vi "Self-Test.vi"(8 "error in (no error)":errorcluster, 11 "VISA resource name":refnum<visa-resource-name>) -> (0 "error out":errorcluster, 1 "Self-Test Result Message":string, 2 "Self-Test Result Code":i32, 3 "VISA resource name out":refnum<visa-resource-name>)   [LabVIEW 2012, in "Micos_uic.lvlib"]
doc: "Runs the instrument's self-test routine and returns the test results."
uses:
  <instrlib>/Micos_uic/Micos_uic.lvlib
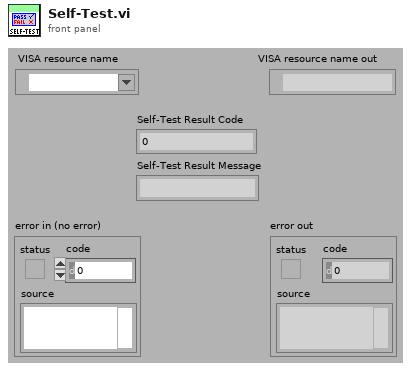
[diagram p1: front panel]
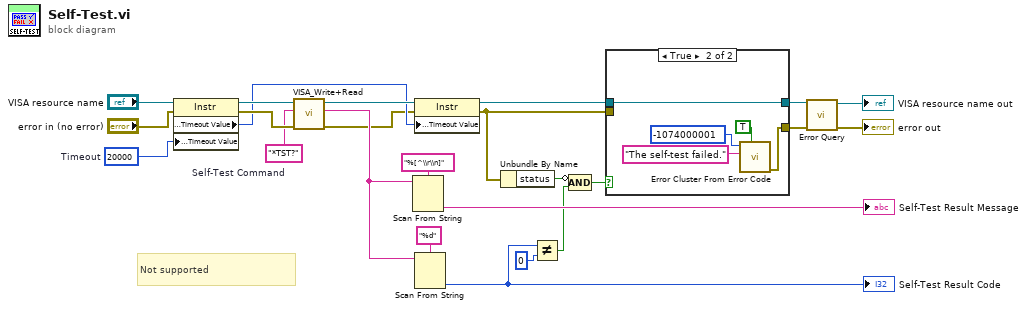
[diagram p0: block diagram]
diagram:
  w16 = u32 20000  # Timeout
  w12 = "*TST?"  # Self-Test Command
  # "Not supported"
  n1 = property class="Instr"(reference="VISA resource name", error in="error in (no error)", "General Settings:Timeout Value"=w16) -> (reference out=w14:refnum<visa-resource-name>, error out=w15:errorcluster, "General Settings:Timeout Value"=w13:u32)
  n2 = call <instrlib>:"VISA_Write+Read.vi"("error in (no error)"=w15, "Write Buffer"=w12, "VISA resource name"=w14) -> ("error out"=w1:errorcluster, "readout"=w2:string, "VISA resource name out"=w22:refnum<visa-resource-name>)  [unwired: 6 in]
  n3 = Scan From String(format string="%[^\\r\\n]" ("Format String"), input string=w2) -> (output 1=→"Self-Test Result Message":string)  [unwired: 3 in, 3 out]
  n4 = property class="Instr"(reference=w22, error in=w1, "General Settings:Timeout Value"=w13) -> (reference out=w11:refnum<visa-resource-name>, error out=w10:errorcluster)
  n5 = Scan From String(format string="%d", input string=w2) -> (output 1=w4:i32)  [unwired: 3 in, 3 out]
  "Self-Test Result Code" <- w4
  n6 = Unbundle By Name(w10) -> ("status"=w6:bool)
  n7 = Not Equal?(x=w4, y=0) -> (x != y?=w7:bool)
  n8 = Compound Arithmetic op=AND(invert w6, w7) -> (w5:bool)
  n9 = case shown="True" w5 {
    tunnel: w11 -> [w26 w31]
    tunnel: w10 -> [w25 _]
    tunnel: [w25 w27] -> w9
    tunnel: [w26 w31] -> w8
    frame False {
    }
    frame True {
      n10 = call <vilib>:"Error Cluster From Error Code.vi"("show call chain? (False)"=TRUE, "error message (\"\")"="The self-test failed." ("Source (VI Name)"), "error code (0)"=-1074000001 ("Code")) -> ("error out"=w27:errorcluster)  [unwired: 6 in]
    }
  }
  n11 = call <instrlib>:"Error Query.vi"("error in (no error)"=w9, "VISA resource name"=w8) -> ("error out"=→"error out":errorcluster, "VISA resource name out"=→"VISA resource name out":refnum<visa-resource-name>)  [unwired: 6 in, 2 out]
